vi "Dataset Types 2 Volts.vi"(7 "Hold":T1, 10 "Dataset Type":T2=enum."Actuator Command") -> (2 "Volts Array":bool[](array[boolean]))   [LabVIEW 2009]
uses:
  Dataset Type.ctl
  Apps/Yes No Button.ctl
panel:
  in  "Volt  Types":T2[](array[typedef])=[enum."Actuator Command", enum."LVDT", enum."Load Cell", enum."Servo Error"]
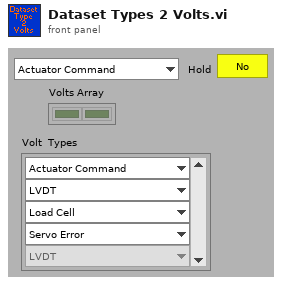
[diagram p1: front panel]
types:
  T1 = typedef "Yes No Button.ctl" = bool
  T2 = typedef "Dataset Type.ctl" = enum16{"LVDT", "Load Cell", "Actuator Command", "Servo Error", "Displacement Command", "Displacement", "Force"}
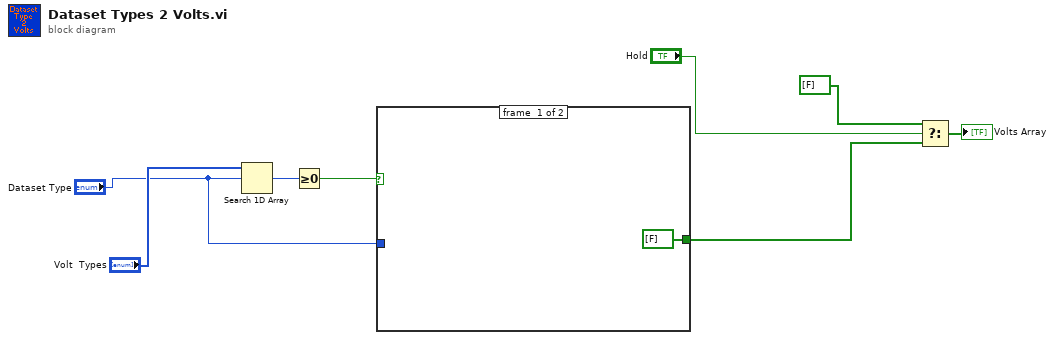
[diagram p0: block diagram]
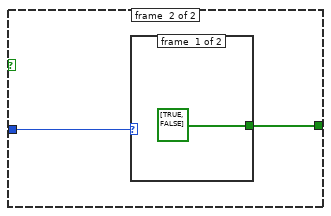
[diagram p2: hidden frame]
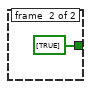
[diagram p3: hidden frame]
diagram:
  n1 = Search 1D Array(1D array="Volt  Types", element="Dataset Type") -> (index of element=w7:i32)  [unwired: 1 in]
  n2 = Greater Or Equal To 0?(x=w7) -> (x >= 0?=w6:bool)
  n3 = case shown="False" w6 {
    tunnel: "Dataset Type" -> [_ w11]
    tunnel: [bool[] [FALSE] ("Volts Array") w10] -> w4
    frame #0 {
    }
    frame #1 {
      n4 = case shown="\"LVDT\", Default" w11 {
        tunnel: [bool[] [TRUE, FALSE] ("Volts Array") bool[] [TRUE] ("Volts Array")] -> w10
        frame #0 {
        }
        frame #1 {
        }
      }
    }
  }
  n5 = Select(t=bool[] [FALSE] ("Volts Array"), s="Hold", f=w4) -> (s? t:f=→"Volts Array":bool[])
